vi "Read Local Resource.vi"(8 "error in (no error)":errorcluster, 11 "6512 in":refnum<class "6512.lvclass">) -> (0 "error out":errorcluster, 2 "Local Resource":refnum<k21>, 3 "6512 out":refnum<class "6512.lvclass">)   [LabVIEW 2019, in "6512.lvlib" / "6512.lvclass"]
uses:
  Library/6512.lvclass
  Library/6512.lvclass/6512.ctl
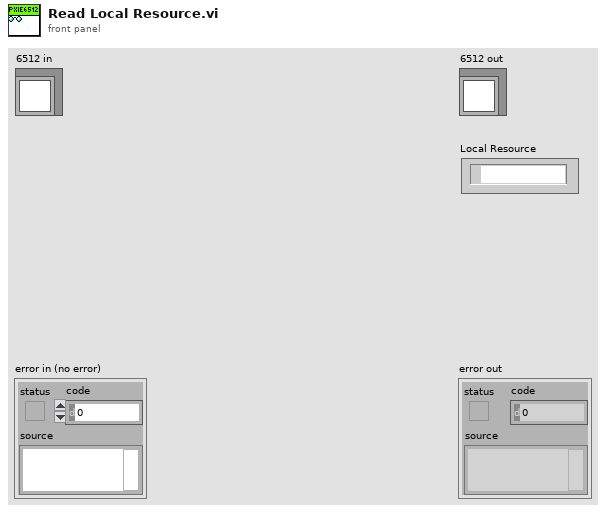
[diagram p1: front panel]
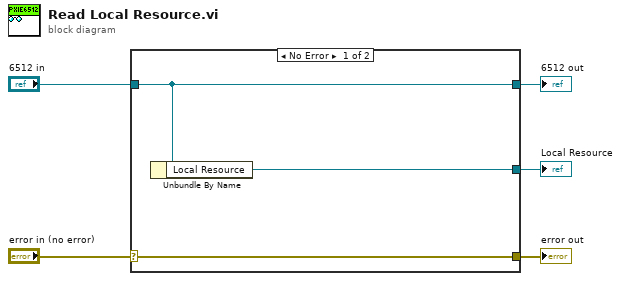
[diagram p0: block diagram]
diagram:
  n1 = case shown="No Error" "error in (no error)" {
    selector: "error in (no error)" -> [w8 w9]
    tunnel: [w8 w9] -> w4
    tunnel: [w7 w10] -> w2
    tunnel: "6512 in" -> [w7 w10]
    tunnel: [w6 _] -> w1
    frame No Error {
      n2 = Unbundle By Name(w7) -> ("Local Resource"=w6:refnum<k21>)
    }
    frame Error {
    }
  }
  "error out" <- w4
  "6512 out" <- w2
  "Local Resource" <- w1
